vi "透明背景.vi"() -> ()   [LabVIEW 2019]
uses:
  User32.dll
panel:
  in  "reference":refnum<vi>
  out "错误输出":errorcluster
  in  "错误输入（无错误）":errorcluster
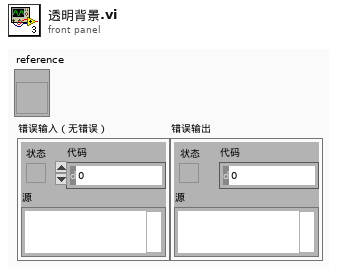
[diagram p1: front panel]
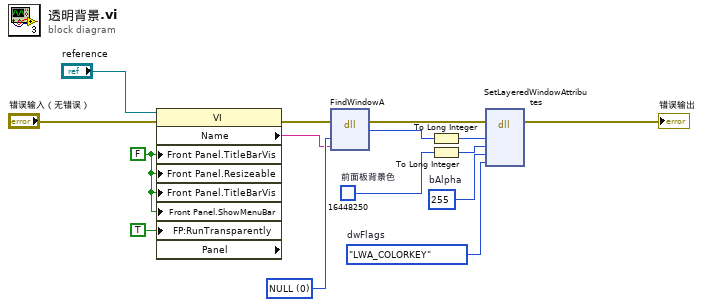
[diagram p0: block diagram]
diagram:
  w4 = FALSE
  w6 = u32 16448250  # 前面板背景色
  w11 = u8 255  # bAlpha
  w9 = enum16{"NONE", "LWA_COLORKEY", "LWA_ALPHA"}."LWA_COLORKEY"  # dwFlags
  w15 = 0 items=["NULL"]
  n1 = property class="VI" props=["Name", "Front Panel.TitleBarVis", "Front Panel.Resizeable", "Front Panel.TitleBarVis", "Front Panel.ShowMenuBar", "FP:RunTransparently", "Panel"](reference="reference", error in="错误输入（无错误）", "Front Panel.TitleBarVis"=w4, "Front Panel.Resizeable"=w4, "Front Panel.TitleBarVis"=w4, "Front Panel.ShowMenuBar"=w4, "FP:RunTransparently"=TRUE) -> (error out=w12:errorcluster, "Name"=w14:string)  [unwired: 2 out]
  n2 = dll-call lib="user32.dll" fn="FindWindowA" label="FindWindow"(error in=w12, "lpszClassName"=w15, "lpszWindowName"=w14) -> (error out=w8:errorcluster, "hWnd"=w13:u32)  [unwired: 4 in, 1 out]
  n3 = To Long Integer(number=w13) -> (32bit integer=w10:i32)
  n4 = To Long Integer(number=w6) -> (32bit integer=w5:i32)
  n5 = dll-call lib="user32.dll" fn="SetLayeredWindowAttributes" label="SetLayeredWindowAttributs"(error in=w8, "handle"=w10, "crkey"=w5, "bAlpha"=w11, "dwFlags"=w9) -> (error out=→"错误输出":errorcluster)  [unwired: 4 in, 4 out]
